vi "MEMR-Optimize Analysis Window.vi"(0 "Gain spectra":cluster{"Freq (Hz)":dbl[], "Mag":dbl[][]}[](array[cluster]), 5 "Threshold":T1, 7 "Noise spectra":cluster{"Freq (Hz)":dbl[], "Mag (dB)":dbl[]}[](array[cluster]), 9 "Level":dbl[](array[numeric])) -> (8 "Fpeak":dbl[](array[numeric]))   [LabVIEW 2020]
uses:
  MEMR-Offline Analysis Parameters.ctl
  Utility VIs/Math VIs/LinSpace (start-stop-step).vi
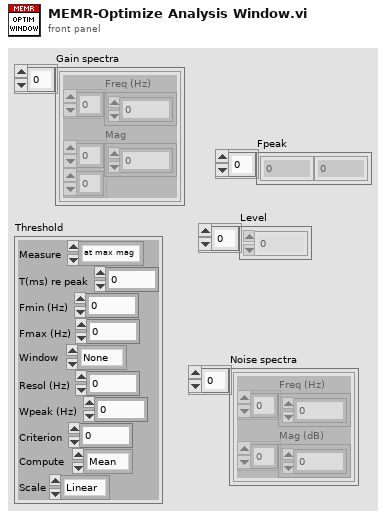
[diagram p1: front panel]
types:
  T1 = typedef "MEMR-Offline Analysis Parameters.ctl" = cluster{"Measure":enum16{"at max mag", "at max gain", "over window", "optimize", "Keefe"}, "T(ms) re peak":dbl, "Fmin (Hz)":dbl, "Fmax (Hz)":dbl, "Window":enum16{"None", "Hanning", "Hamming"}, "Resol (Hz)":dbl, "Wpeak (Hz)":dbl, "Criterion":dbl, "Compute":enum16{"Mean", "Sum"}, "Scale":enum16{"Linear", "Log"}}
  T2 = enum16{"at max mag", "at max gain", "over window", "optimize", "Keefe"}
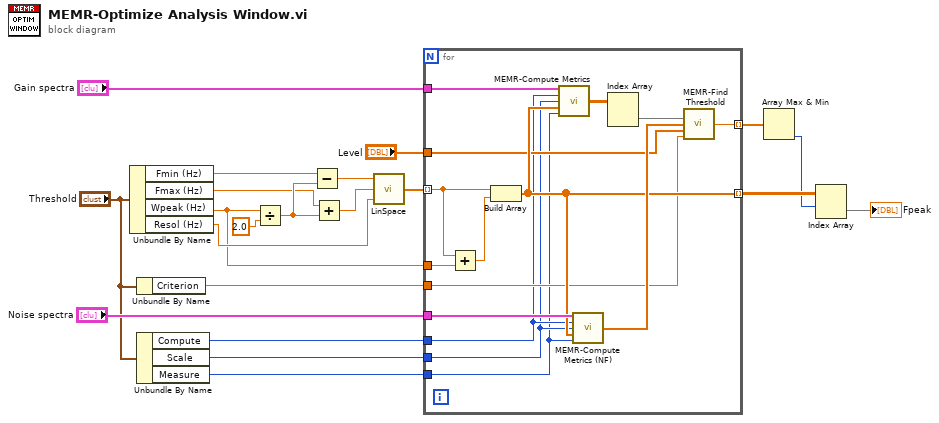
[diagram p0: block diagram]
diagram:
  n1 = Unbundle By Name("Threshold") -> ("Fmin (Hz)"=w18:dbl, "Fmax (Hz)"=w16:dbl, "Wpeak (Hz)"=w6:dbl, "Resol (Hz)"=w7:dbl)
  n2 = Unbundle By Name("Threshold") -> ("Criterion"=w5:dbl)
  n3 = Unbundle By Name("Threshold") -> ("Compute"=w3:enum16{"Mean", "Sum"}, "Scale"=w2:enum16{"Linear", "Log"}, "Measure"=w1:T2)
  n4 = Divide(x=w6, y=2.0) -> (x/y=w17:dbl)
  n5 = Subtract(x=w18, y=w17) -> (x-y=w15:dbl)
  n6 = Add(x=w16, y=w17) -> (x+y=w14:dbl)
  n7 = call-poly "LinSpace.vi"("Step"=w7, "Stop"=w14, "Start"=w15) -> ("Array"=w13:dbl[])  [unwired: 1 in, 1 out]
  n8 = for {
    tunnel: "Noise spectra" -> [w36]
    tunnel: "Gain spectra" -> [w35]
    tunnel: w13 -> [w33] mode=indexing
    tunnel: w6 -> [w34]
    tunnel: [w28] -> w11 mode=indexing
    tunnel: [w27] -> w12 mode=indexing
    tunnel: "Level" -> [w26]
    tunnel: w5 -> [w25]
    tunnel: w3 -> [w24]
    tunnel: w2 -> [w23]
    tunnel: w1 -> [w22]
    n9 = Add(x=w33, y=w34) -> (x+y=w32:dbl)
    n10 = Build Array(w33, w32) -> (w28:dbl[])
    n11 = call "MEMR-Compute Metrics.vi"("Gain spectra in"=w35, "Compute"=w24, "Scale"=w23, "Fpeak"=w28, "Measure"=w22) -> ("Metrics"=w31:dbl[][])  [unwired: 9 in, 1 out]
    n12 = call "MEMR-Compute Metrics (NF).vi"("Gain spectra in"=w36, "Compute"=w24, "Scale"=w23, "Fpeak"=w28, "Measure"=w22) -> ("Metrics"=w29:dbl[])  [unwired: 9 in, 1 out]
    n13 = Index Array(array=w31) -> (element=w30:dbl[])  [unwired: 2 in]
    n14 = call "MEMR-Find Threshold.vi"("Metrics"=w30, "Noise"=w29, "Level"=w26, "Criterion"=w25) -> ("Threshold"=w27:dbl)  [unwired: 11 in]
  }
  n15 = Array Max & Min(array=w12) -> (min index (indices)=w10:i32)  [unwired: 3 out]
  n16 = Index Array(array=w11, index (row)=w10) -> (element=→"Fpeak":dbl[])  [unwired: 1 in]
